vi "IsInsideExample.vi"() -> ()   [LabVIEW 2010]
uses:
  <vilib>/vision/NI_Vision_Development_Module.lvlib
panel:
  out "Img":T1(plugin-control)
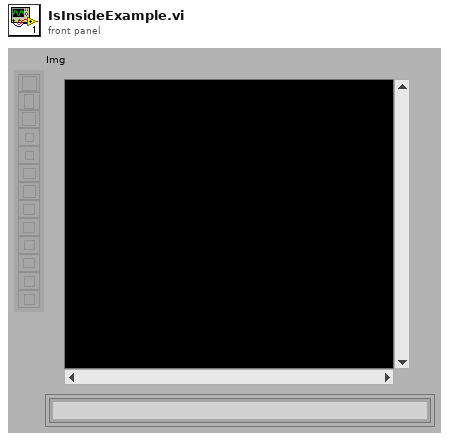
[diagram p1: front panel]
types:
  T1 = typedef "IMAQ Image.ctl" = refnum<image>
  T2 = cluster{"Area":dbl, "Number of Holes":dbl, "Bounding Rect":cluster{"Left":dbl, "Top":dbl, "Right":dbl, "Bottom":dbl}, "Center of Mass":cluster{"X":dbl, "Y":dbl}, "Orientation":dbl, "Dimensions":cluster{"Width":dbl, "Height":dbl}}[]
  T3 = cluster{"Global Rectangle":i32[], "Contours":cluster{"Contour Type":u32, "ROI Type":u32, "Points":i32[]}[]}
  T4 = typedef "ROI Descriptor" = cluster{"Global Rectangle":i32[], "Contours":cluster{"ID":enum32{"External", "Internal"}, "Type":u32, "Coordinates":i32[]}[]}
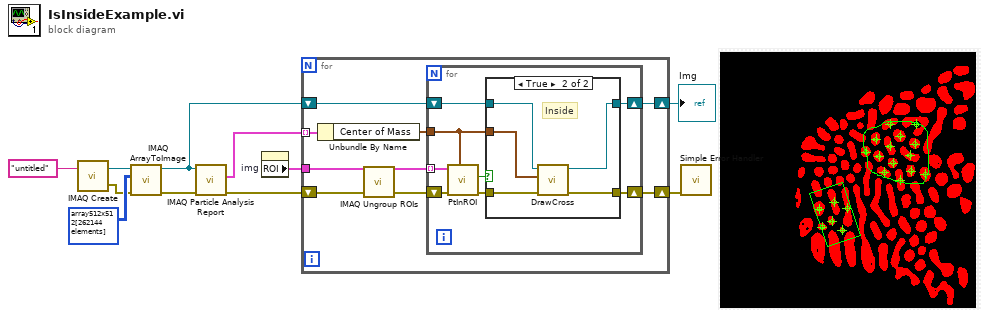
[diagram p0: block diagram]
diagram:
  n1 = call "IMAQ Create"("Image Name"="untitled") -> ("New Image"=w6:T1, "error out"=w4:errorcluster)  [unwired: 4 in]
  n2 = call "IMAQ ArrayToImage"("error in (no error)"=w4, "Image Pixels (U8)"=u8[][] array512x512[262144 elements], "Image"=w6) -> ("error out"=w3:errorcluster, "Image Out"=w5:T1)  [unwired: 7 in]
  n3 = call "IMAQ Particle Analysis Report"("error in (no error)"=w3, "Image"=w5) -> ("error out"=w2:errorcluster, "Particle Reports (Pixels)"=w10:T2)  [unwired: 4 in, 4 out]
  n4 = property on="img" class="ImageControl"() -> ("ROI"=w11:T3)  [unwired: 2 in, 2 out]
  n5 = for {
    tunnel: w11 -> [w15]
    tunnel: w10 -> [w20] mode=indexing
    shift-right: [w18] -> w9
    shift-left: w5 -> [w19]
    shift-right: [w17] -> w1
    shift-left: w2 -> [w13]
    n6 = Unbundle By Name(w20) -> ("Center of Mass"=w16:cluster{"X":dbl, "Y":dbl})
    n7 = call "IMAQ Ungroup ROIs"("error in (no error)"=w13, "ROI Descriptor"=w15) -> ("error out"=w12:errorcluster, "ROI Descriptors out"=w14:T4[])  [unwired: 2 in]
    n8 = for {
      tunnel: w16 -> [w21]
      tunnel: w14 -> [w22] mode=indexing
      shift-right: [w24] -> w17
      shift-left: w12 -> [w25]
      shift-right: [w27] -> w18
      shift-left: w19 -> [w28]
      n9 = call "PtInROI.vi"("Point"=w21, "error in (no error)"=w25, "ROI Descriptor In"=w22) -> ("error out"=w26:errorcluster, "IsInside"=w23:bool)  [unwired: 7 in]
      n10 = case shown="True" w23 {
        tunnel: w28 -> [w29 w34]
        tunnel: w21 -> [_ w30]
        tunnel: [w29 w33] -> w27
        tunnel: w26 -> [_ w32]
        tunnel: [_ w31] -> w24
        frame False {
        }
        frame True {
          # "Inside"
          n11 = call "DrawCross.vi"("error out 2"=w32, "Center"=w30, "Image In"=w34) -> ("error out"=w31:errorcluster, "Image Out"=w33:T1)  [unwired: 7 in]
        }
      }
    }
  }
  "Img" <- w9
  n12 = call <vilib>:"Simple Error Handler.vi"("error in (no error)"=w1) -> ()  [unwired: 4 in, 5 out]
